vi "Get Motor IO Refnum.vi"(8 "error in (no error)":errorcluster, 11 "SGDV_Ctrl_Class in":refnum<class "SGDV Motor.lvclass">) -> (0 "error out":errorcluster, 2 "Motor IO Refnum":T1={"SEN"="A/AO0", "PWM"="A/PWM0", "SIGN (Vel Dir)"="A/DIO0", "Enc"="A/ENC", "SON"="B/DIO0", "CLR"="A/DIO0", "S-RDY"="C/DIO5", "ALM"="A/DIO3", "ALM-RST"="A/DIO6", "ALO1"="B/DIO1", "ALO2"="B/DIO2", "ALO3"="B/DIO3"}, 3 "SGDV_Ctrl_Class out":refnum<class "SGDV Motor.lvclass">)   [LabVIEW 2013, in "SGDV_Ctrl_v13_lib.lvlib" / "SGDV Motor.lvclass"]
uses:
  SGDV Motor.lvclass
  Controls and General VIs/Motor IO Refnum.ctl
  SGDV Motor.lvclass/SGDV Motor.ctl
  SGDV_Ctrl_v13_lib.lvlib
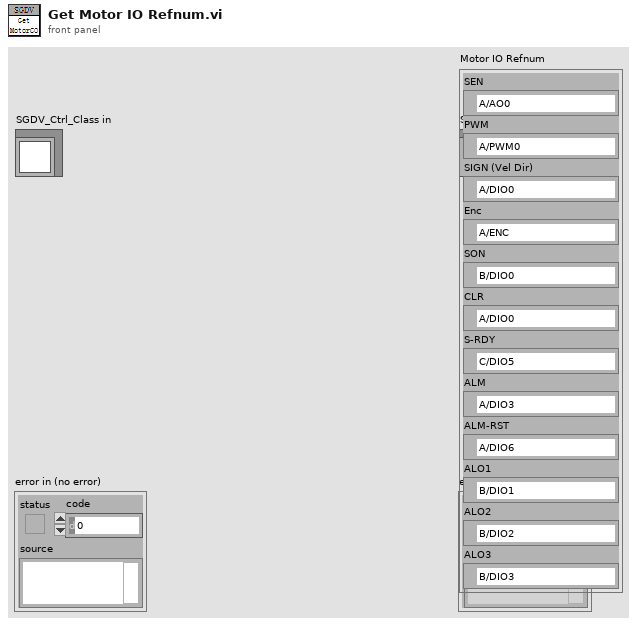
[diagram p1: front panel]
types:
  T1 = typedef "SGDV_Ctrl_v13_lib.lvlib/Motor IO Refnum.ctl" = cluster{"SEN":tag, "PWM":tag, "SIGN (Vel Dir)":tag, "Enc":tag, "SON":tag, "CLR":tag, "S-RDY":tag, "ALM":tag, "ALM-RST":tag, "ALO1":tag, "ALO2":tag, "ALO3":tag}
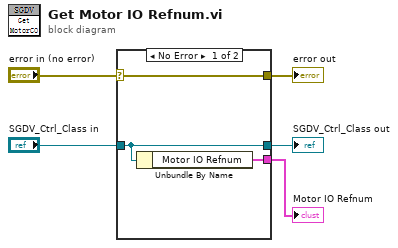
[diagram p0: block diagram]
diagram:
  n1 = case shown="No Error" "error in (no error)" {
    selector: "error in (no error)" -> [w8 w9]
    tunnel: [w8 w9] -> w4
    tunnel: [w7 w10] -> w2
    tunnel: "SGDV_Ctrl_Class in" -> [w7 w10]
    tunnel: [w6 _] -> w1
    frame No Error {
      n2 = Unbundle By Name(w7) -> ("Motor IO Refnum"=w6:T1)
    }
    frame Error {
    }
  }
  "error out" <- w4
  "SGDV_Ctrl_Class out" <- w2
  "Motor IO Refnum" <- w1
